vi "TestDBConnection.vi"() -> ()   [LabVIEW 2015]
uses:
  CustomControl/UserRight.ctl
  <vilib>/addons/database/Connection.llb/DB Tools Open Connec (String).vi
  <vilib>/addons/database/NI_Database_API.lvlib
panel:
  out "error out 2":errorcluster
  in  "ID_Number":string="1111"
  out "UserRight":T1
  out "Message":string
  out "error out":errorcluster
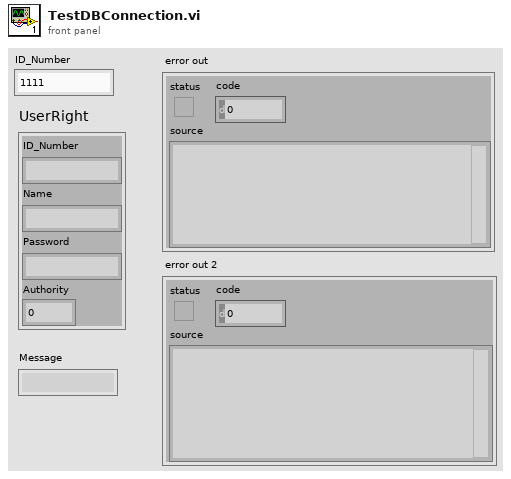
[diagram p1: front panel]
types:
  T1 = typedef "UserRight.ctl" = cluster{"ID_Number":string, "Name":string, "Password":string, "Authority":i32}
  T2 = typedef "NI_Database_API.lvlib/Conn ObjectReference.ctl" = refnum<k1>
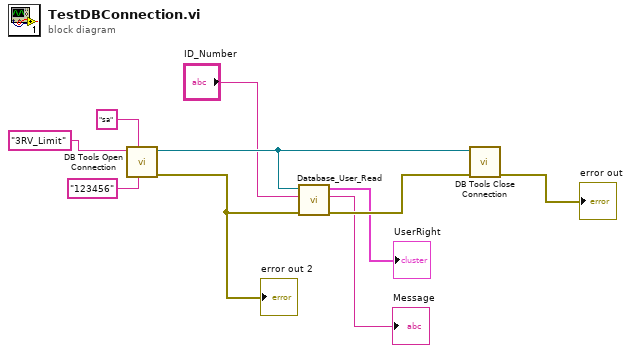
[diagram p0: block diagram]
diagram:
  n1 = call-poly <vilib>:"DB Tools Open Connection.vi"("password"="123456", "userID"="sa", "connection information"="3RV_Limit" ("userID")) -> ("error out"=w6:errorcluster, "connection reference"=w4:T2)  [unwired: 5 in]
  "error out 2" <- w6
  n2 = call "Database_User_Read.vi"("error in"=w6, "ID_Number"="ID_Number", "connection reference"=w4) -> ("error out"=w5:errorcluster, "Message"=→"Message":string, "UserRight"=→"UserRight":T1)  [unwired: 5 in, 1 out]
  n3 = call <vilib>:"DB Tools Close Connection.vi"("error in (no error)"=w5, "connection reference"=w4) -> ("error out"=→"error out":errorcluster)  [unwired: 5 in]
